vi "test Get Message Status Channels.vi"(8 "error in":errorcluster, 11 "TestCase in":refnum<class "Scripting.lvclass">) -> (0 "error out":errorcluster, 3 "TestCase out":refnum<class "Scripting.lvclass">)   [LabVIEW 2020, in "Scripting.lvclass"]
uses:
  Scripting.lvclass
  C:/Git/niveristand-custom-device-testing-tools/VeriStandScriptingTestCase/VeriStandScriptingTestCase.lvclass
  Shared/1553 Channel.ctl
  Shared/Address.ctl
  Shared/Message Definition.ctl
  Shared/Message Type.ctl
  Shared/Terminal Endpoint.ctl
  Shared/Parameter Definition.ctl
  niveristand-custom-device-testing-tools/VeriStandScriptingTestCase/VeriStandScriptingTestCase.lvclass/VeriStandScriptingTestCase.ctl
  niveristand-custom-device-testing-tools/VeriStandScriptingTestCase/Read Target.vi
  NationalInstruments.VeriStand.SystemDefinitionAPI
  <vilib>/addons/_JKI Toolkits/VI Tester/TestCase.llb/TestCase.lvclass
  Scripting/Ballard MIL-STD-1553 Scripting.lvlib
  C:/Program Files (x86)/National Instruments/LabVIEW 2020/vi.lib/addons/_JKI Toolkits/VI Tester/TestCase.llb/TestCase.lvclass
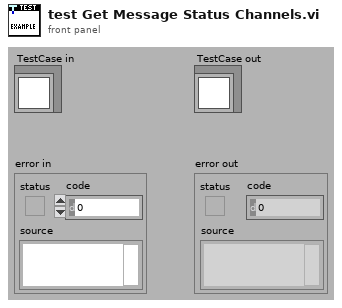
[diagram p1: front panel]
types:
  T1 = typedef "1553 Channel.ctl" = cluster{"HW channel":u16, "terminal addresses":T2[], "acyclic frame names":string[], "messages":T3[]}
  T2 = typedef "Address.ctl" = u16
  T3 = typedef "Message Definition.ctl" = cluster{"name":string, "message type":T4, "endpoint Tx":T5, "endpoint Rx":T5, "create timestamp channel":bool, "mode code":u16, "number of words":u16, "parameters":cluster{"name":string, "default value":dbl, "unit":string, "parameter definition":T6}[]}
  T4 = typedef "Message Type.ctl" = string
  T5 = typedef "Terminal Endpoint.ctl" = cluster{"terminal address":T2, "subaddress":T2}
  T6 = typedef "Parameter Definition.ctl" = cluster{"start index":i32, "size (bits)":i32, "encoding":enum16{"BNR", "BCD", "Discrete"}, "signed":bool, "multiplier":dbl, "offset":dbl}
  T7 = typedef "Custom Device API.lvlib/Custom Device Item Ref.ctl" = u64
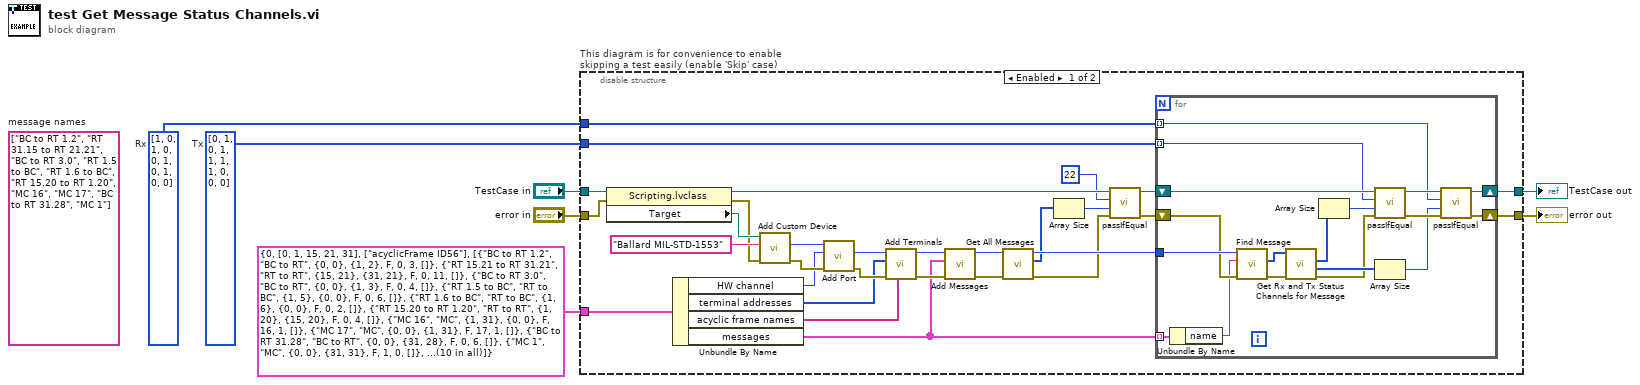
[diagram p0: block diagram]
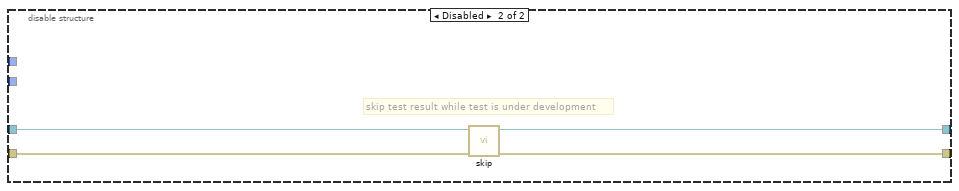
[diagram p2: hidden frame]
diagram:
  w2 = i32[] [1, 0, 1, 0, 0, 1, 0, 1, 0, 0]  # Rx
  w1 = i32[] [0, 1, 0, 1, 1, 1, 1, 0, 0, 0]  # Tx
  (unwired) string[] ["BC to RT 1.2", "RT 31.15 to RT 21.21", "BC to RT 3.0", "RT 1.5 to BC", "RT 1.6 to BC", "RT 15.20 to RT 1.20", "MC 16", "MC 17", "BC to RT 31.28", "MC 1"]  # message names
  n1 = disable-structure "This diagram is for convenience to enable skipping a test easily (enable 'Skip' case)" shown="Enabled" {
    disable-tunnel: "TestCase in" -> [w36 w59]
    disable-tunnel: [w15 w57] -> w4
    disable-tunnel: [w12 w58] -> w6
    disable-tunnel: "error in" -> [w9 w56]
    disable-tunnel: T1 {"HW channel"=0, "terminal addresses"=[0, 1, 15, 21, 31], "acyclic frame names"=["acyclicFrame ID56"], "messages"=[{"name"="BC to RT 1.2", "message type"="BC to RT", "endpoint Tx"={"terminal address"=0, "subaddress"=0}, "endpoint Rx"={"terminal address"=1, "subaddress"=2}, "create timestamp channel"=FALSE, "mode code"=0, "number of words"=3, "parameters"=[]}, {"name"="RT 15.21 to RT 31.21", "message type"="RT to RT", "endpoint Tx"={"terminal address"=15, "subaddress"=21}, "endpoint Rx"={"terminal address"=31, "subaddress"=21}, "create timestamp channel"=FALSE, "mode code"=0, "number of words"=11, "parameters"=[]}, {"name"="BC to RT 3.0", "message type"="BC to RT", "endpoint Tx"={"terminal address"=0, "subaddress"=0}, "endpoint Rx"={"terminal address"=1, "subaddress"=3}, "create timestamp channel"=FALSE, "mode code"=0, "number of words"=4, "parameters"=[]}, {"name"="RT 1.5 to BC", "message type"="RT to BC", "endpoint Tx"={"terminal address"=1, "subaddress"=5}, "endpoint Rx"={"terminal address"=0, "subaddress"=0}, "create timestamp channel"=FALSE, "mode code"=0, "number of words"=6, "parameters"=[]}, {"name"="RT 1.6 to BC", "message type"="RT to BC", "endpoint Tx"={"terminal address"=1, "subaddress"=6}, "endpoint Rx"={"terminal address"=0, "subaddress"=0}, "create timestamp channel"=FALSE, "mode code"=0, "number of words"=2, "parameters"=[]}, {"name"="RT 15.20 to RT 1.20", "message type"="RT to RT", "endpoint Tx"={"terminal address"=1, "subaddress"=20}, "endpoint Rx"={"terminal address"=15, "subaddress"=20}, "create timestamp channel"=FALSE, "mode code"=0, "number of words"=4, "parameters"=[]}, {"name"="MC 16", "message type"="MC", "endpoint Tx"={"terminal address"=1, "subaddress"=31}, "endpoint Rx"={"terminal address"=0, "subaddress"=0}, "create timestamp channel"=FALSE, "mode code"=16, "number of words"=1, "parameters"=[]}, {"name"="MC 17", "message type"="MC", "endpoint Tx"={"terminal address"=0, "subaddress"=0}, "endpoint Rx"={"terminal address"=1, "subaddress"=31}, "create timestamp channel"=FALSE, "mode code"=17, "number of words"=1, "parameters"=[]}, {"name"="BC to RT 31.28", "message type"="BC to RT", "endpoint Tx"={"terminal address"=0, "subaddress"=0}, "endpoint Rx"={"terminal address"=31, "subaddress"=28}, "create timestamp channel"=FALSE, "mode code"=0, "number of words"=6, "parameters"=[]}, {"name"="MC 1", "message type"="MC", "endpoint Tx"={"terminal address"=0, "subaddress"=0}, "endpoint Rx"={"terminal address"=31, "subaddress"=31}, "create timestamp channel"=FALSE, "mode code"=1, "number of words"=0, "parameters"=[]}]} ("1553 channel") -> [w13 _]
    disable-tunnel: w2 -> [w11 _]
    disable-tunnel: w1 -> [w10 _]
    frame Enabled {
      n2 = property class="Scripting.lvclass"(reference=w36, error in=w9) -> (reference out=w23:refnum<class "Scripting.lvclass">, error out=w8:errorcluster, "Target"=w35:refnum<k24>)
      n3 = Unbundle By Name(w13) -> ("HW channel"=w31:u16, "terminal addresses"=w26:T2[], "acyclic frame names"=w25:string[], "messages"=w20:T3[])
      n4 = call "Add Custom Device.vi"("error in"=w8, "name"="Ballard MIL-STD-1553", "target in"=w35) -> ("error out"=w34:errorcluster, "Ballard MIL-STD 1553 custom device"=w33:T7)  [unwired: 6 in, 1 out]
      n5 = call "Add Port.vi"("error in"=w34, "port number"=w31, "Ballard MIL-STD 1553 custom device in"=w33) -> ("error out"=w29:errorcluster, "port"=w30:T7)  [unwired: 6 in, 1 out]
      n6 = call "Add Terminals.vi"("acyclic frame names"=w25, "error in"=w29, "terminal addresses"=w26, "port in"=w30) -> ("error out"=w27:errorcluster, "port out"=w28:T7)  [unwired: 6 in]
      n7 = call "Add Messages.vi"("error in"=w27, "messages"=w20, "port in"=w28) -> ("error out"=w24:errorcluster, "port out"=w32:T7)  [unwired: 7 in]
      n8 = call "Get All Messages.vi"("error in"=w24, "port in"=w32) -> ("error out"=w18:errorcluster, "messages"=w16:T7[], "port out"=w21:T7)  [unwired: 7 in]
      n9 = Array Size(array=w16) -> (size(s)=w22:i32)
      n10 = call-dynamic "passIfEqual.vi"("error in (no error)"=w18, "y"=w22, "x"=22 ("size(s)"), "TestCase in"=w23) -> ("error out"=w17:errorcluster, "TestCase out"=w14:refnum<class "Scripting.lvclass">)  [unwired: 6 in]
      n11 = for {
        shift-right: [w38] -> w12
        shift-left: w17 -> [w54]
        tunnel: w20 -> [w53] mode=indexing
        shift-right: [w50] -> w15
        shift-left: w14 -> [w49]
        tunnel: w21 -> [w55]
        tunnel: w10 -> [w45] mode=indexing
        tunnel: w11 -> [w43] mode=indexing
        n12 = Unbundle By Name(w53) -> ("name"=w40:string)
        n13 = call "Find Message.vi"("error in"=w54, "message name"=w40, "port in"=w55) -> ("error out"=w52:errorcluster, "message refs"=w46:T7[])  [unwired: 5 in, 2 out]
        n14 = call "Get Rx and Tx Status Channels for Message.vi"("error in"=w52, "message refs"=w46) -> ("error out"=w39:errorcluster, "Rx status channels"=w44:T7[], "Tx status channels"=w47:T7[])  [unwired: 6 in, 1 out]
        n15 = Array Size(array=w47) -> (size(s)=w42:i32)
        n16 = call-dynamic "passIfEqual.vi"("error in (no error)"=w39, "y"=w42, "x"=w45, "TestCase in"=w49) -> ("error out"=w51:errorcluster, "TestCase out"=w48:refnum<class "Scripting.lvclass">)  [unwired: 6 in]
        n17 = Array Size(array=w44) -> (size(s)=w41:i32)
        n18 = call-dynamic "passIfEqual.vi"("error in (no error)"=w51, "y"=w41, "x"=w43, "TestCase in"=w48) -> ("error out"=w38:errorcluster, "TestCase out"=w50:refnum<class "Scripting.lvclass">)  [unwired: 6 in]
      }
    }
    frame Disabled {
      # "skip test result while test is under development"
      n19 = call <vilib>:"skip.vi"("error in (no error)"=w56, "TestCase in"=w59) -> ("error out"=w58:errorcluster, "TestCase out"=w57:refnum<class "Scripting.lvclass">)  [unwired: 8 in]
    }
  }
  "error out" <- w6
  "TestCase out" <- w4
